vi "FTW-STR-Array-Delimit.vi"(5 "Array of Strings":string[](array[string]), 7 "Delimiter":string=",") -> (6 "Delimited String":string)   [LabVIEW 2014]
panel:
  # "Inputs"
  # "Outputs"
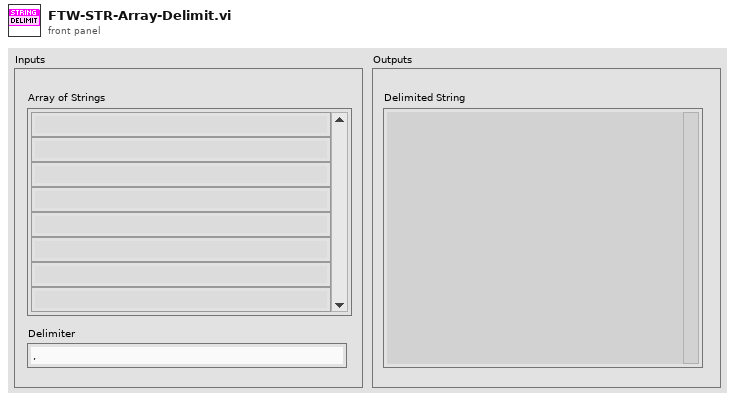
[diagram p1: front panel]
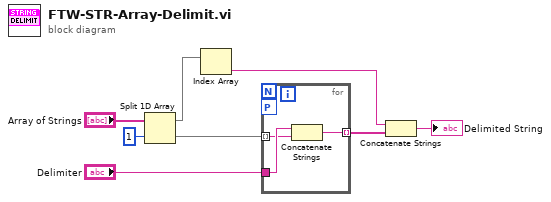
[diagram p0: block diagram]
diagram:
  n1 = Split 1D Array(array="Array of Strings", index=1) -> (first subarray=w5:string[], second subarray=w6:string[])
  n2 = Index Array(array=w5) -> (element=w3:string)  [unwired: 1 in]
  n3 = for {
    tunnel: w6 -> [w10] mode=indexing
    tunnel: "Delimiter" -> [w11]
    tunnel: [w9] -> w2 mode=indexing
    workers-P: _ -> [_]
    n4 = Concatenate Strings(w11, w10) -> (w9:string)
  }
  n5 = Concatenate Strings(w3, w2) -> (→"Delimited String":string)
